vi "Write plugin info.vi"(8 "error in (no error)":errorcluster, 10 "plugin info":T1, 11 "DSFPlugin in":refnum<class "DSFPlugin.lvclass">) -> (0 "error out":errorcluster, 3 "DSFPlugin out":refnum<class "DSFPlugin.lvclass">)   [LabVIEW 2017, in "DSFPlugin.lvclass"]
uses:
  DSFPlugin.lvclass
  Controls/dsf plugin.ctl
  Controls/dsf timing.ctl
  DSFPlugin.lvclass/DSFPlugin.ctl
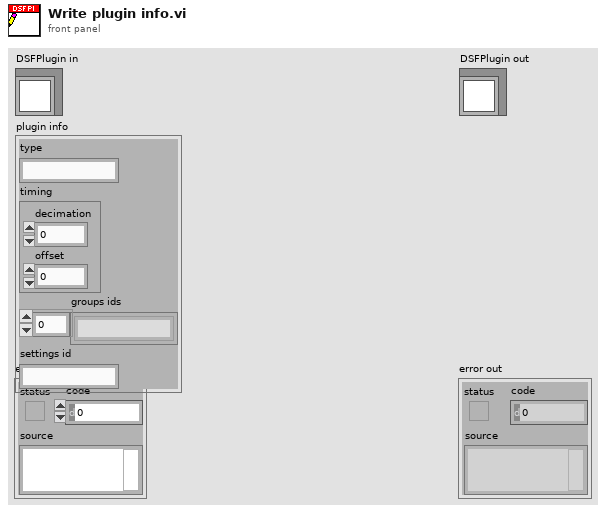
[diagram p1: front panel]
types:
  T1 = typedef "dsf plugin.ctl" = cluster{"type":string, "timing":T2, "groups ids":string[], "settings id":string}
  T2 = typedef "dsf timing.ctl" = cluster{"decimation":i32, "offset":i32}
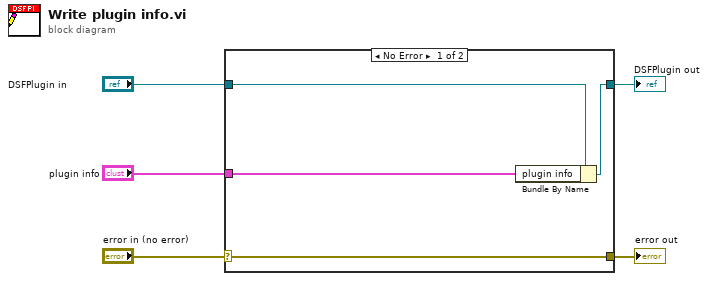
[diagram p0: block diagram]
diagram:
  n1 = case shown="No Error" "error in (no error)" {
    selector: "error in (no error)" -> [w9 w10]
    tunnel: [w9 w10] -> w4
    tunnel: [w7 w11] -> w2
    tunnel: "DSFPlugin in" -> [w8 w11]
    tunnel: "plugin info" -> [w6 _]
    frame No Error {
      n2 = Bundle By Name(cluster=w8, "plugin info"=w6) -> (w7:refnum<class "DSFPlugin.lvclass">)
    }
    frame Error {
    }
  }
  "error out" <- w4
  "DSFPlugin out" <- w2
